vi "Close.vi"(8 "error in (no error)":errorcluster, 11 "Agilent_3458 in":refnum<class "Agilent_3458.lvclass">) -> (0 "error out":errorcluster, 3 "Agilent_3458 out":refnum<class "Agilent_3458.lvclass">)   [LabVIEW 2018, in "DigitizerPlugins.lvlib" / "Agilent_3458.lvclass"]
uses:
  Agilent_3458.lvclass
  C:/ICDAS/NistPluggableModules/Digitizer/DigitizerPlugins/DigitizerBaseClass/DigitizerBase.lvclass
  DigitizerBaseClass/DigitizerBase.lvclass/DigitizerBase.ctl
  DigitizerBaseClass/Accessors/Read Handle.vi
  <instrlib>/Agilent 3458/Agilent 3458.lvlib
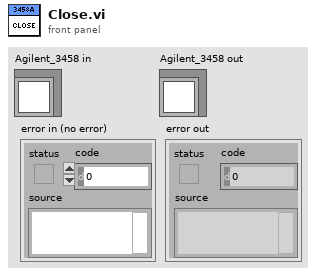
[diagram p1: front panel]
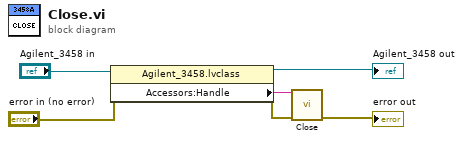
[diagram p0: block diagram]
diagram:
  n1 = property class="Agilent_3458.lvclass"(reference="Agilent_3458 in", error in="error in (no error)") -> (reference out=→"Agilent_3458 out":refnum<class "Agilent_3458.lvclass">, error out=w3:errorcluster, "Accessors:Handle"=w4:string)
  n2 = call <instrlib>:"Close.vi"("error in (no error)"=w3, "VISA resource name"=w4) -> ("error out"=→"error out":errorcluster)  [unwired: 9 in]
